vi "Acquire.vi"(5 "Test State Timer":dbl, 8 "error in (no error)":errorcluster, 9 "Notifiier Data":T3, 10 "notifier out":refnum<notifier>, 11 "Hardware Resources in":T4) -> (0 "error out":errorcluster, 2 "Notifier Data Out":T3, 3 "Averaged Data Array":dbl[](array[numeric]))   [LabVIEW 2026, in "Acquisition.lvlib"]
doc: "Perform the acquisition. Replace the contents of this diagram with calls to acquisition hardware."
uses:
  Acquisition.lvlib
  Hardware Configuration.ctl
  controls/NotifierAndDataQueue.ctl
  controls/WaveformChartData.ctl
  <vilib>/DAQmx/read.llb/DAQmx Read (Analog 2D DBL NChan NSamp).vi
  <vilib>/DAQmx/miscellaneous.llb/DAQmx Fill In Error Info.vi
  <vilib>/DAQmx/read.llb/DAQmx Read (Digital 1D Bool 1Chan 1Samp).vi
  Settings/Settings.lvlib
panel:
  in  "Waveform Chart Data":T1
  out "Waveform Chart":T2(graph)
  out "data":bool[](array[boolean])
  out "Current":dbl
  out "Air Flow":dbl
  out "Dut RPM":dbl
  out "Motor RPM":dbl
  out "ambient Temp":dbl
  out "Dut Temp":dbl
  out "DUT Vacuum":dbl
  out "Tank vacuum":dbl
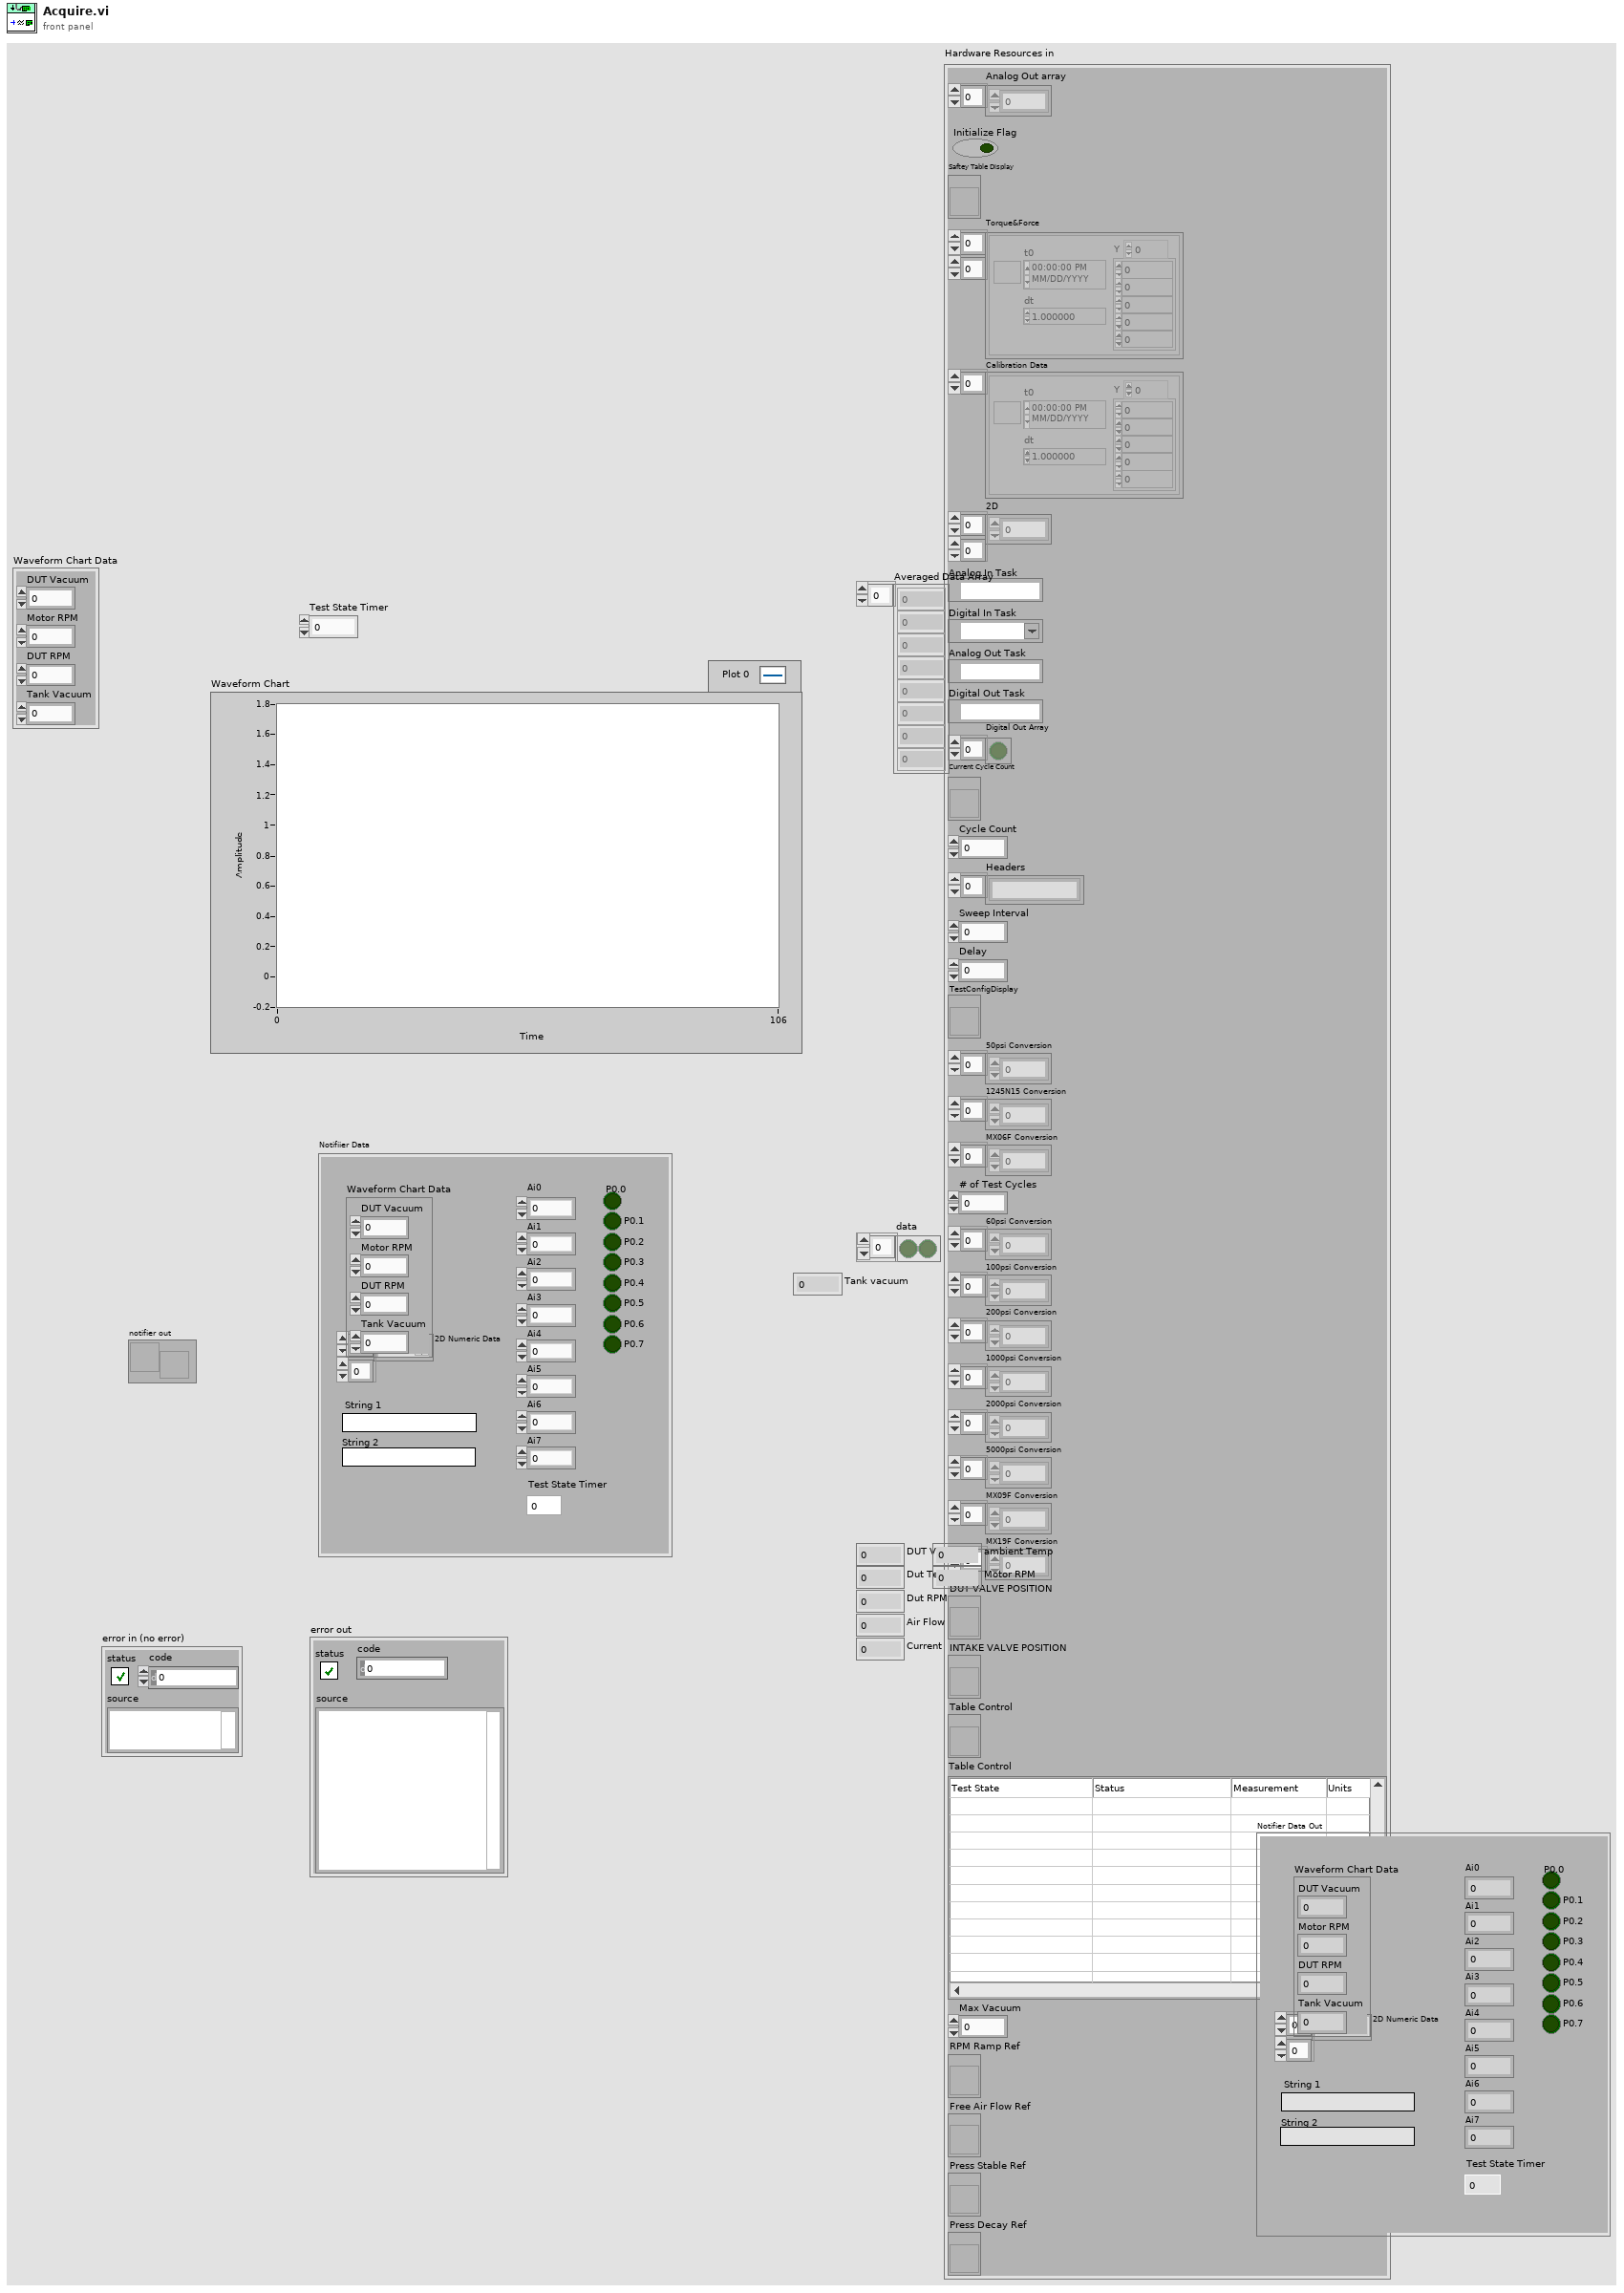
[diagram p1: front panel]
types:
  T1 = typedef "Settings.lvlib/WaveformChartData.ctl" = cluster{"DUT Vacuum":dbl, "Motor RPM":dbl, "DUT RPM":dbl, "Tank Vacuum":dbl}
  T2 = cluster{"DUT Vacuum":dbl, "Motor RPM":dbl, "DUT RPM":dbl, "Tank Vacuum":dbl}
  T3 = typedef "NotifierAndDataQueue.ctl" = cluster{"Ai0":dbl, "Ai1":dbl, "Ai2":dbl, "Ai3":dbl, "Ai4":dbl, "Ai5":dbl, "Ai6":dbl, "Ai7":dbl, "P0.0":bool, "P0.1":bool, "P0.2":bool, "P0.3":bool, "P0.4":bool, "P0.5":bool, "P0.6":bool, "P0.7":bool, "2D Numeric Data":dbl[][], "String 2":string, "String 1":string, "Waveform Chart Data":T1, "Test State Timer":dbl}
  T4 = typedef "Acquisition.lvlib/Hardware Configuration.ctl" = cluster{"Analog Out array":dbl[], "Initialize Flag":bool, "Saftey Table Display":refnum<vi>, "Torque&Force":waveform(dbl)[][], "Calibration Data":waveform(dbl)[], "2D":dbl[][], "Analog In Task":refnum<k21>, "Digital In Task":refnum<k21>, "Analog Out Task":refnum<k21>, "Digital Out Task":refnum<k21>, "Digital Out Array":bool[], "Current Cycle Count":refnum<vi>, "Cycle Count":u64, "Headers":string[], "Sweep Interval":u64, "Delay":u64, "TestConfigDisplay":refnum<vi>, "50psi Conversion":dbl[], "1245N15 Conversion":dbl[], "MX06F Conversion":dbl[], "# of Test Cycles":u64, "60psi Conversion":dbl[], "100psi Conversion":dbl[], "200psi Conversion":dbl[], "1000psi Conversion":dbl[], "2000psi Conversion":dbl[], "5000psi Conversion":dbl[], "MX09F Conversion":dbl[], "MX19F Conversion":dbl[], "DUT VALVE POSITION":refnum<vi>, "INTAKE VALVE POSITION":refnum<vi>, "Table Control":refnum<vi>, "Table Control":string[][], "Max Vacuum":dbl, "RPM Ramp Ref":refnum<vi>, "Free Air Flow Ref":refnum<vi>, "Press Stable Ref":refnum<vi>, "Press Decay Ref":refnum<vi>}
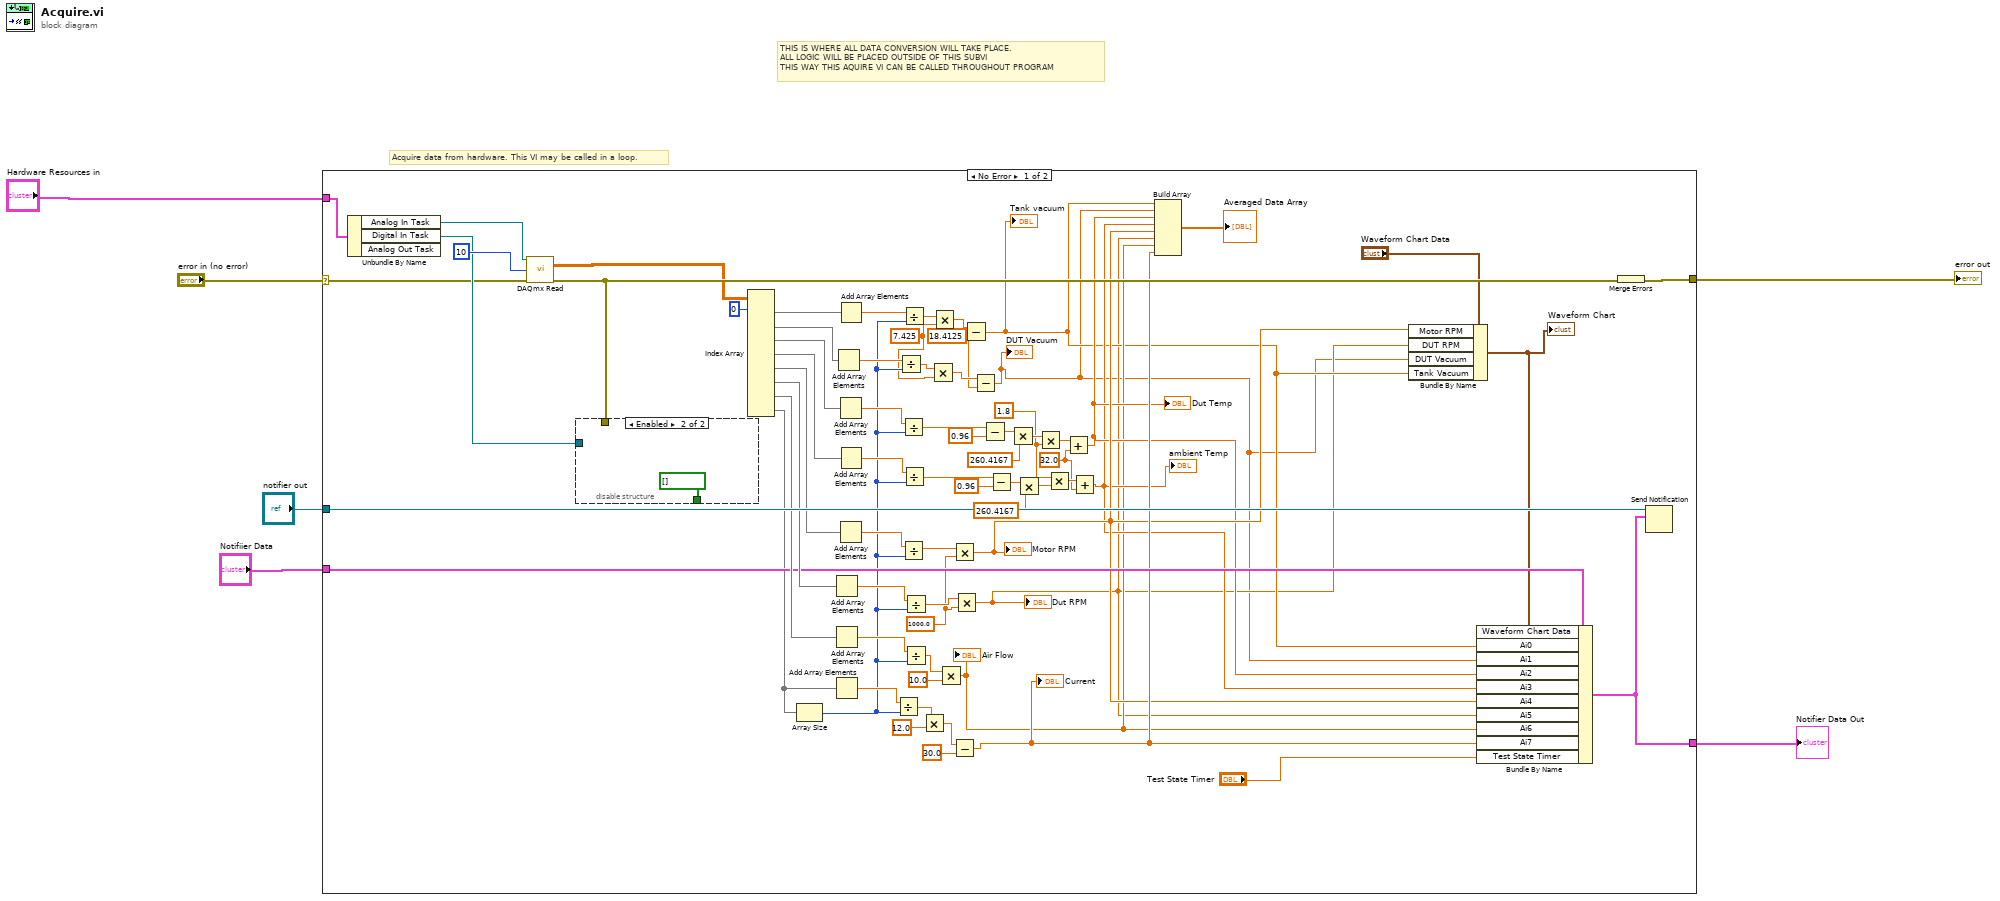
[diagram p0: block diagram]
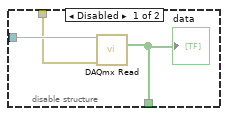
[diagram p2: hidden frame]
diagram:
  # "THIS IS WHERE ALL DATA CONVERSION WILL TAKE PLACE.\nALL LOGIC WILL BE PLACED OUTSIDE OF THIS SUBVI\nTHIS WAY THIS AQUIRE VI CAN BE CALLED THROUGHOUT PROGRAM"
  # "Acquire data from hardware. This VI may be called in a loop."
  n1 = case shown="No Error" "error in (no error)" {
    selector: "error in (no error)" -> [w54 w82]
    tunnel: [w76 w82] -> w5
    tunnel: "Hardware Resources in" -> [w62 _]
    tunnel: "notifier out" -> [w75 _]
    tunnel: [w52 w81] -> w2
    tunnel: "Notifiier Data" -> [w51 w81]
    frame No Error {
      w16 = 32.0
      w19 = 1.8 ("y")
      w30 = 18.4125 ("y")
      w31 = 7.425 ("y")
      w36 = 1000.0 ("y")
      n2 = Unbundle By Name(w62) -> ("Analog In Task"=w61:refnum<k21>, "Digital In Task"=w55:refnum<k21>)  [unwired: 1 out]
      n3 = call-poly <vilib>:"DAQmx Read.vi"("task/channels in"=w61, "number of samples per channel"=10, "error in"=w54) -> ("data"=w50:dbl[][], "error out"=w53:errorcluster)  [unwired: 10 in, 1 out]
      n4 = disable-structure shown="Enabled" {
        disable-tunnel: w55 -> [w79 _]
        disable-tunnel: [w78 bool[] [] ("data")] -> _
        disable-tunnel: w53 -> [w77 _]
        frame Disabled {
          n5 = call-poly <vilib>:"DAQmx Read.vi"("task/channels in"=w79, "error in"=w77) -> ("data"=w78:bool[])  [unwired: 11 in, 2 out]
          "data" <- w78
        }
        frame Enabled {
        }
      }
      n6 = Index Array(array=w50, index (row) #1=0 ("index (row)")) -> (element #1=w67:dbl[], element #2=w69:dbl[], element #3=w72:dbl[], element #4=w66:dbl[], element #5=w65:dbl[], element #6=w64:dbl[], element #7=w63:dbl[], element #8=w49:dbl[])  [unwired: 15 in]
      n7 = Array Size(array=w49) -> (size(s)=w48:i32)
      n8 = Add Array Elements(numeric array=w64) -> (sum=w58:dbl)
      n9 = Add Array Elements(numeric array=w63) -> (sum=w57:dbl)
      n10 = Add Array Elements(numeric array=w49) -> (sum=w56:dbl)
      n11 = Add Array Elements(numeric array=w69) -> (sum=w71:dbl)
      n12 = Add Array Elements(numeric array=w72) -> (sum=w74:dbl)
      n13 = Add Array Elements(numeric array=w65) -> (sum=w59:dbl)
      n14 = Add Array Elements(numeric array=w67) -> (sum=w68:dbl)
      n15 = Add Array Elements(numeric array=w66) -> (sum=w60:dbl)
      n16 = Divide(x=w56, y=w48) -> (x/y=w29:dbl)
      n17 = Divide(x=w71, y=w48) -> (x/y=w32:dbl)
      n18 = Divide(x=w74, y=w48) -> (x/y=w46:dbl)
      n19 = Divide(x=w59, y=w48) -> (x/y=w38:dbl)
      n20 = Divide(x=w68, y=w48) -> (x/y=w35:dbl)
      n21 = Divide(x=w60, y=w48) -> (x/y=w39:dbl)
      n22 = Divide(x=w58, y=w48) -> (x/y=w37:dbl)
      n23 = Divide(x=w57, y=w48) -> (x/y=w12:dbl)
      n24 = Multiply(x=w29, y=12.0) -> (x*y=w28:dbl)
      n25 = Multiply(x=w32, y=w31) -> (x*y=w33:dbl)
      n26 = Multiply(x=w35, y=w31) -> (x*y=w34:dbl)
      n27 = Multiply(x=w12, y=10.0) -> (x*y=w11:dbl)
      "Air Flow" <- w11
      n28 = Multiply(x=w38, y=w36) -> (x*y=w24:dbl)
      "Motor RPM" <- w24
      n29 = Subtract(x=w28, y=30.0) -> (x-y=w27:dbl)
      "Current" <- w27
      n30 = Multiply(x=w37, y=w36) -> (x*y=w8:dbl)
      "Dut RPM" <- w8
      n31 = Subtract(x=w34, y=w30) -> (x-y=w9:dbl)
      "Tank vacuum" <- w9
      n32 = Subtract(x=w33, y=w30) -> (x-y=w7:dbl)
      "DUT Vacuum" <- w7
      n33 = Subtract(x=w46, y=0.96) -> (x-y=w44:dbl)
      n34 = Subtract(x=w39, y=0.96) -> (x-y=w41:dbl)
      n35 = Multiply(x=w44, y=260.4167) -> (x*y=w21:dbl)
      n36 = Multiply(x=w41, y=260.4167) -> (x*y=w20:dbl)
      n37 = Multiply(x=w21, y=w19) -> (x*y=w18:dbl)
      n38 = Multiply(x=w19, y=w20) -> (x*y=w17:dbl)
      n39 = Add(x=w18, y=w16) -> (x+y=w15:dbl)
      "Dut Temp" <- w15
      n40 = Add(x=w17, y=w16) -> (x+y=w14:dbl)
      "ambient Temp" <- w14
      n41 = Build Array(w9, w7, w15, w14, w24, w8, w11, w27) -> (→"Averaged Data Array":dbl[])
      n42 = Bundle By Name(cluster="Waveform Chart Data", "Motor RPM"=w24, "DUT RPM"=w8, "DUT Vacuum"=w7, "Tank Vacuum"=w9) -> (w22:T1)
      "Waveform Chart" <- w22
      n43 = Bundle By Name(cluster=w51, "Waveform Chart Data"=w22, "Ai0"=w9, "Ai1"=w7, "Ai2"=w15, "Ai3"=w14, "Ai4"=w24, "Ai5"=w8, "Ai6"=w11, "Ai7"=w27, "Test State Timer"="Test State Timer") -> (w52:T3)
      n44 = Merge Errors(w53) -> (w76:errorcluster)
      n45 = Send Notification(notification=w52, notifier=w75) -> ()  [unwired: 1 in, 2 out]
    }
    frame Error {
    }
  }
  "error out" <- w5
  "Notifier Data Out" <- w2
